vi "Waveform_Extract from Start and End Index.vi"(8 "Error":errorcluster, 9 "End Index\n(-1) Last point":i32, 10 "Start Index":i32, 11 "Raw Data Waveform":T1) -> (0 "Error Out":errorcluster, 1 "End Out":i32, 2 "Start Out":i32, 3 "Waveform Out":T1)   [LabVIEW 2016]
doc: "Retrieves a subset of a waveform at a specified time or index. You must manually select the polymorphic instance you want to use."
uses:
  Universal Controls/Waveform_Data.ctl
  Universal Controls/Read Write Button.ctl
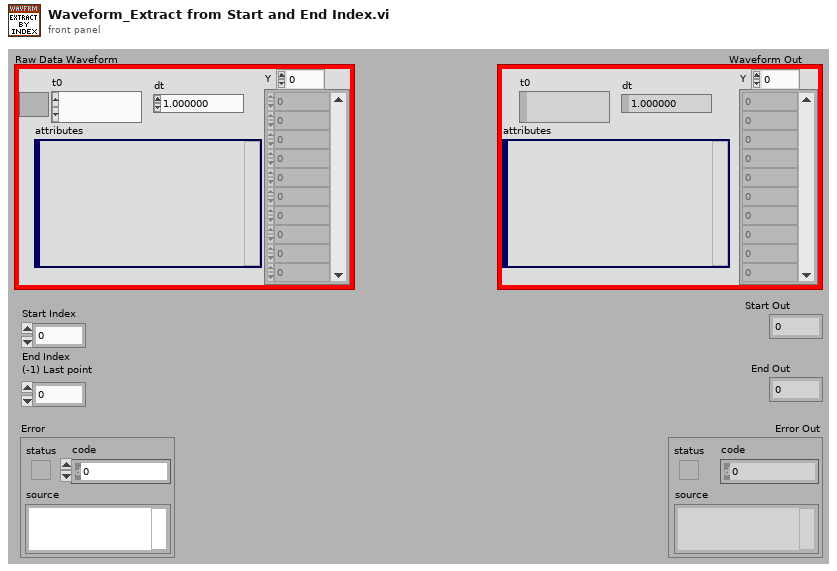
[diagram p1: front panel]
types:
  T1 = typedef "Waveform_Data.ctl" = waveform(dbl)
  T2 = typedef "Read Write Button.ctl" = bool
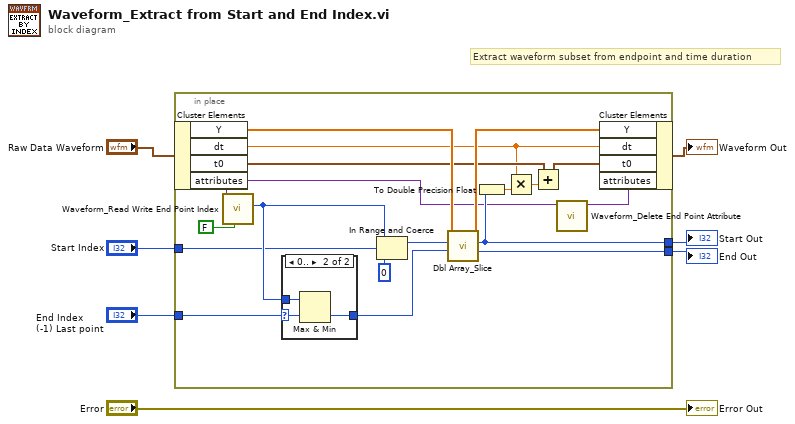
[diagram p0: block diagram]
diagram:
  # "Extract waveform subset from endpoint and time duration"
  n1 = in-place {
    in-place-border: [w17] -> w4
    in-place-border: [w20] -> w3
    in-place-border: "Start Index" -> [w13]
    in-place-border: "End Index\n(-1) Last point" -> [w11]
    n2 = in-place-cluster #1("Raw Data Waveform") -> ("Y"=w25:dbl[], "dt"=w19:dbl, "t0"=w22:timestamp, "attributes"=w9:variant)
    n3 = call "Waveform_Read Write End Point Index.vi"("Read(f)\nWrite(t)"=T2 FALSE ("Read(f)\nWrite(t)"), "Waveform Atributes"=w9) -> ("End Point Out"=w14:i32)  [unwired: 7 in, 2 out]
    n4 = case shown="0.." w11 {
      selector: w11 -> [_ w29]
      tunnel: w14 -> [w26 w28]
      tunnel: [w26 w27] -> w10
      frame ..-1 {
      }
      frame 0.. {
        n5 = Max & Min(x=w28, y=w29) -> (min(x,y)=w27:i32)  [unwired: 1 out]
      }
    }
    n6 = In Range and Coerce(upper limit=w14, x=w13, lower limit=0) -> (coerced(x)=w12:i32)  [unwired: 1 out]
    n7 = call "Dbl Array_Slice.vi"("End Index\n(-1) Last point"=w10, "Start Index"=w12, "Array"=w25) -> ("End Out"=w20:i32, "Start Out"=w17:i32, "Subarray (array[i:j]) Out"=w24:dbl[])  [unwired: 1 in, 5 out]
    n8 = To Double Precision Float(number=w17) -> (double precision float=w18:dbl)
    n9 = Multiply(x=w19, y=w18) -> (x*y=w23:dbl)
    n10 = Add(x=w22, y=w23) -> (x+y=w21:timestamp)
    n11 = call "Waveform_Delete End Point Attribute.vi"("Waveform Atributes"=w9) -> ("Waveform Atributes Out"=w8:variant)  [unwired: 9 in, 1 out]
    n12 = in-place-cluster #1("Y"=w24, "dt"=w19, "t0"=w21, "attributes"=w8) -> (→"Waveform Out":T1)
  }
  "Start Out" <- w4
  "End Out" <- w3
  "Error Out" <- "Error"
